vi "Configure Normalize.vi"(6 "Store Trace As Refer.(F: Disable)":bool, 7 "Enable Normalize (T: Enable)":bool=TRUE, 8 "error in (no error)":errorcluster, 9 "Normalized Reference Position (10)":dbl=10.0, 10 "Normalized Reference Level (0 dB)":dbl, 11 "VISA resource name":refnum<visa-resource-name>) -> (0 "error out":errorcluster, 3 "VISA resource name out":refnum<visa-resource-name>)   [LabVIEW 2022 SP3, in "Agilent N934X Series.lvlib"]
doc: "Configures the normalize function. This VI is functional only when Measurement Type has been set to Tracking Generator."
uses:
  <instrlib>/Agilent N934X Series/Agilent N934X Series.lvlib
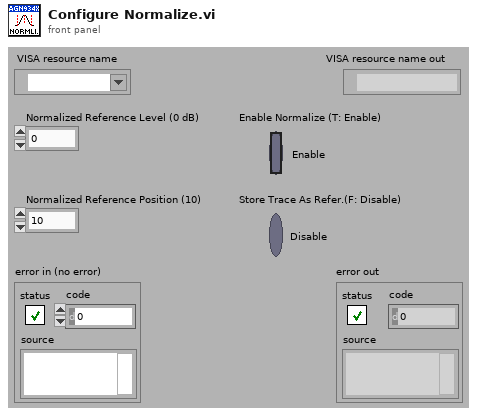
[diagram p1: front panel]
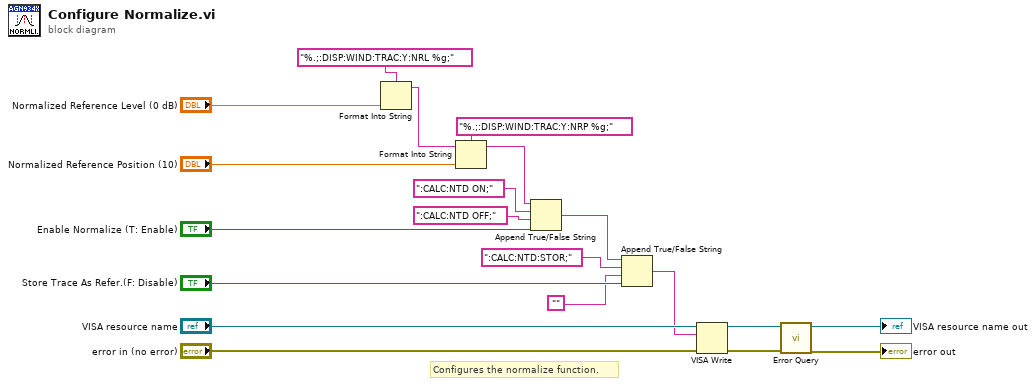
[diagram p0: block diagram]
diagram:
  # "Configures the normalize function."
  n1 = Format Into String(format string="%.;:DISP:WIND:TRAC:Y:NRL %g;", "Normalized Reference Level (0 dB)") -> (resulting string=w18:string)  [unwired: 2 in, 1 out]
  n2 = Format Into String(format string="%.;:DISP:WIND:TRAC:Y:NRP %g;", initial string=w18, "Normalized Reference Position (10)") -> (resulting string=w15:string)  [unwired: 1 in, 1 out]
  n3 = Append True/False String(1:"Enable Normalize (T: Enable)", 2:":CALC:NTD OFF;", 3:":CALC:NTD ON;", 4:w15) -> (0:w4:string)
  n4 = Append True/False String(1:"Store Trace As Refer.(F: Disable)", 2:"", 3:":CALC:NTD:STOR;", 4:w4) -> (0:w2:string)
  n5 = VISA Write(VISA resource name="VISA resource name", write buffer=w2, error in (no error)="error in (no error)") -> (VISA resource name out=w10:refnum<visa-resource-name>, error out=w9:errorcluster)  [unwired: 1 out]
  n6 = call <instrlib>:"Error Query.vi"("error in (no error)"=w9, "VISA resource name"=w10) -> ("error out"=→"error out":errorcluster, "VISA resource name out"=→"VISA resource name out":refnum<visa-resource-name>)  [unwired: 6 in, 2 out]
